vi "8-channel 24-bit TDM Transmit.vi"() -> ()   [LabVIEW 2013]
uses:
  <vilib>/Platform/TimedLoop/XDataNode/timing_clust.ctl
  <vilib>/Platform/TimedLoop/XDataNode/nitl_modes.ctl
  <vilib>/Platform/TimedLoop/XDataNode/wakeup.ctl
  Source/Controls/transmitter configuration.ctl
  Source/Controls/sync modes.ctl
  <vilib>/rvi/DataTransferAndStorage/Container/Common/niFpgaContainerGetUniqueNameForEmu.vi
  <vilib>/rvi/DataTransferAndStorage/Container/Common/niFpgaContainerSetEmuInfo.vi
  <vilib>/rvi/eio/common/nirviEmuReportErrorAndStop.vi
  <vilib>/rvi/Emulation/niFpgaSctlEmulationGetInTimedLoop.vi
  <vilib>/rvi/Emulation/niFpgaEmulationReportErrorSimple.vi
  <vilib>/rvi/Emulation/niFpgaGetClockAttributes.vi
  <vilib>/rvi/DataTransferAndStorage/Container/Common/niFpgaContainerExecOnDevCompGetState.vi
  <vilib>/rvi/FIFO/Fifo_Resource/nirvififoEmulationWriteFpgaImpl.vi
  <vilib>/rvi/interface/RandomDataEmulation/nirviRandomDataFPGAFIFO.vi
  <vilib>/rvi/interface/RandomDataEmulation/niFpgaRandomDataHandleErrors.vi
  <vilib>/rvi/Emulation/niFpgaCriticalErrorInLSC.vi
  <vilib>/rvi/FIFO/Fifo_Resource/nirvififoEmulationReadFpgaImpl.vi
  <vilib>/rvi/FIFO/Fifo_Resource/nirvififoEmulationGetNumberOfElementsToReadFpgaImpl.vi
  <vilib>/Platform/TimedLoop/XDataNode/XDataNode.xnode
  <vilib>/rvi/LocalResourceManager/LocalResourceManager.xnode
  <vilib>/rvi/DataTransferAndStorage/Container/XNode/niFpgaContainer.xnode
  <vilib>/rvi/FIFO/Fifo_Resource/niFpgaFifoEmulationRefIn.vi
  <vilib>/Platform/TimedLoop/XDataNode/XDNodeRunTimeDep.lvlib
  Source/I2S-TDM.lvlib
panel:
  out "FIFO Elements":u32
  out "signals out":cluster{"clock":bool, "sync":bool, "sdata":bool}
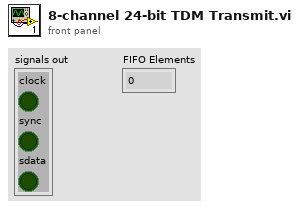
[diagram p1: front panel]
types:
  T1 = typedef "XDNodeRunTimeDep.lvlib/timing_clust.ctl" = cluster{"Expected End [f-1]":u64, "Actual End [f-1]":u64, "Finished Late? [f-1]":bool, "Expected End [i-1]":u64, "Actual End [i-1]":u64, "Finished Late? [i-1]":bool, "Expected Start [i]":u64, "Actual Start [i]":u64, "Expected Start [f]":u64, "Actual Start [f]":u64, "Source Name":string, "Structure Name":string, "Period":i64, "Deadline":i64, "Offset":i64, "Start":i64, "Priority":i32, "Timeout":i32, "Mode":T2, "Wakeup Reason":T3, "Error":errorcluster, "Source Type":string, "Secondary Source Type":string, "Global End Time":u64, "Global Start Time":u64, "Frame Duration":u64, "Iteration Duration":u64, "Assigned CPU":i32, "I/O Scan Engine Mode":u32}
  T2 = typedef "XDNodeRunTimeDep.lvlib/nitl_modes.ctl" = enum32{"No Change", "Process missed periods, maintain original phase", "Discard missed periods, maintain original phase", "Process missed periods, ignore original phase", "Discard missed periods, ignore original phase"}
  T3 = typedef "XDNodeRunTimeDep.lvlib/wakeup.ctl" = enum32{"Normal", "Aborted", "Asynchronous wakeup", "Timing source error", "Timed loop error", "Timeout"}
  T4 = typedef "I2S-TDM.lvlib/transmitter configuration.ctl" = cluster{"number of channels":u8, "bits per channel":u8, "data set edge":enum16{"rising", "falling"}, "sync mode":T5, "invert sync":bool}
  T5 = typedef "I2S-TDM.lvlib/sync modes.ctl" = enum16{"TDM - Sample Clock", "TDM - Pre-Start Pulse"}
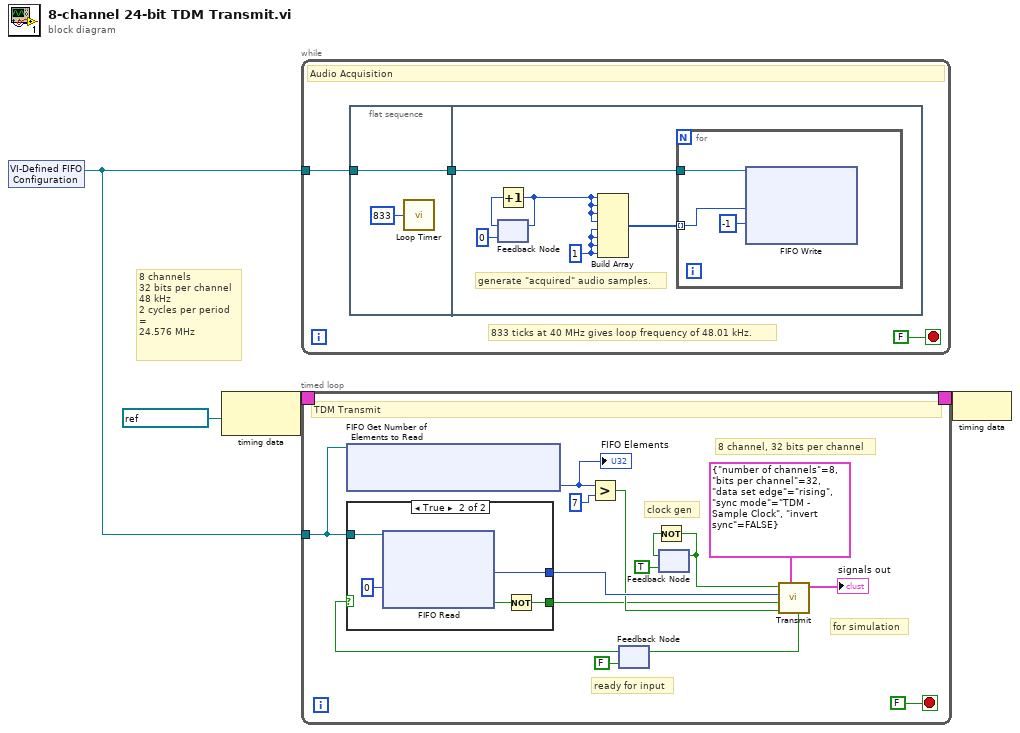
[diagram p0: block diagram]
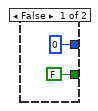
[diagram p2: hidden frame]
diagram:
  # "8 channels\n32 bits per channel\n48 kHz\n2 cycles per period\n=\n24.576 MHz"
  n1 = xnode "VI-Defined FIFO Configuration"() -> ("FIFO Out"=w1:refnum<k21>)
  n2 = node-c288(refnum<k21> "24.576MHz" ("Source Name")) -> (w4:T1)
  n3 = while {
    tunnel: w1 -> [w7]
    stop <- FALSE stop-if-true
    # "833 ticks at 40 MHz gives loop frequency of 48.01 kHz."
    # "Audio Acquisition"
    n4 = flat-sequence {
      tunnel: w7 -> [w9]
      tunnel: [w9] -> w6
      tunnel: w6 -> [w15]
      frame #0 {
        n5 = call "Loop Timer"("Count(Ticks)"=u16 833) -> ()  [unwired: 1 out]
      }
      frame #1 {
        w10 = u32 1
        # "generate \"acquired\" audio samples."
        n6 = feedback #1(u32 0) -> (w14:u32)
        n7 = Increment(x=w14) -> (x+1=w12:u32)
        n8 = feedback-in #1(w12) -> ()
        n9 = Build Array(w12, w12, w12, w12, w10, w10, w10, w10) -> (w11:u32[])
        n10 = for {
          tunnel: w15 -> [w18]
          tunnel: w11 -> [w17] mode=indexing
          n11 = xnode ("FIFO Write")("Element"=w17, "Timeout"=-1, "FIFO In"=w18) -> ()  [unwired: 2 out]
        }
      }
    }
  }
  n12 = timed-loop {
    timing: w4 -> [_]
    timing-out: [_] -> w3
    tunnel: w1 -> [w33]
    stop <- FALSE stop-if-true
    # "clock gen"
    # "8 channel, 32 bits per channel"
    # "for simulation"
    # "ready for input"
    # "TDM Transmit"
    n13 = xnode ("FIFO Get Number of Elements to Read")("FIFO In"=w33) -> ("Number of Elements to Read"=w32:u32)  [unwired: 1 out]
    "FIFO Elements" <- w32
    n14 = Greater?(x=w32, y=u32 7) -> (0:w23:bool)
    n15 = feedback #2(FALSE ("ready for input")) -> (w25:bool)
    n16 = case shown="True" w25 {
      tunnel: w33 -> [_ w40]
      tunnel: [u32 0 ("Element") w39] -> w28
      tunnel: [FALSE w36] -> w21
      frame False {
      }
      frame True {
        n17 = xnode ("FIFO Read")("Timeout"=0, "FIFO In"=w40) -> ("Element"=w39:u32, "Timed Out?"=w37:bool)  [unwired: 1 out]
        n18 = Not(x=w37) -> (.not. x?=w36:bool)
      }
    }
    n19 = feedback #3(TRUE) -> (w30:bool)
    n20 = Not(x=w30) -> (.not. x?=w19:bool)
    n21 = feedback-in #3(w19) -> ()
    n22 = call "Transmit.vi"("configuration"=T4 {"number of channels"=8, "bits per channel"=32, "data set edge"=enum."rising", "sync mode"=enum."TDM - Sample Clock", "invert sync"=FALSE}, "transmit"=w23, "input valid"=w21, "sample"=w28, "clock in"=w19) -> ("signals out"=→"signals out":cluster{"clock":bool, "sync":bool, "sdata":bool}, "ready for input"=w27:bool)  [unwired: 5 in]
    n23 = feedback-in #2(w27) -> ()
  }
  n24 = node-c288(w3) -> ()
